vi "PH_gentec_P-Link.Action Measure.vi"(0 "VI in":refnum<vi>, 5 "error in (no error)":errorcluster) -> (14 "VI out":refnum<vi>, 19 "error out":errorcluster)   [LabVIEW 2014, in "PH_gentec_P-Link.lvlib"]
uses:
  PH_gentec_P-Link.lvlib
  PH_Basics/PH_Powermeter_BaseClass/PH_Powermeter_BaseClass.State.ctl
  PH_Basics/PH_Powermeter_BaseClass/PH_Powermeter_BaseClass.lvlib
  instr.lib/Gentec-P-Link/gentec-P-Link - Driver.lvlib
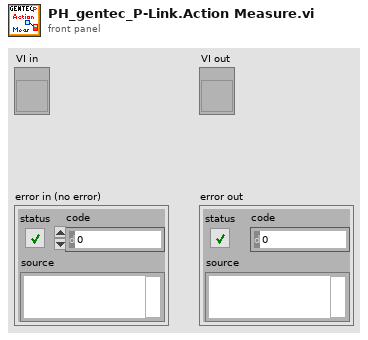
[diagram p1: front panel]
types:
  T1 = typedef "PH_Powermeter_BaseClass.lvlib/PH_Powermeter_BaseClass.State.ctl" = enum32{"off", "operating", "opened", "checked", "connected", "Sets to change", "running"}
  T2 = typedef "PH_Powermeter_BaseClass.lvlib/PH_Powermeter_BaseClass.i attribute.ctl" = cluster{"GUI References":T3, "Connection":T4, "Head Attributes":T5, "VISA resource":refnum<visa-resource-name>, "Energy":T6, "Service ID Energy":i32, "Wanted Settings":T7, "Current Settings":T7}
  T3 = typedef "PH_Powermeter_BaseClass.lvlib/PH_Powermeter_BaseClass.GUI Refs.ctl" = cluster{"Head Attributes":refnum<vi>, "Energy":refnum<vi>, "Connection":refnum<vi>, "VISA Resource":refnum<vi>, "Scaling Factor":refnum<vi>, "Range":refnum<vi>, "Wavelength":refnum<vi>, "Trigger Level":refnum<vi>, "Wanted Settings":refnum<vi>, "Current Settings":refnum<vi>}
  T4 = typedef "PH_Powermeter_BaseClass.lvlib/PH_Powermeter_BaseClass.Connection.ctl" = cluster{"failed checks":i8, "Timeout":bool, "Data read":string, "Failure":bool, "Error":bool, "State":T1}
  T5 = typedef "PH_Powermeter_BaseClass.lvlib/PH_Powermeter_BaseClass.Head Attributes.ctl" = cluster{"Instrument Type":string, "Head Version":string, "Head Name":string, "Serial Number":string, "Firmware":string, "Sensor Type":string, "MinimumRange":u32, "Maximum Range":u32, "Min Wavelength":i32, "Max Wavelength":i32}
  T6 = typedef "PH_Powermeter_BaseClass.lvlib/PH_Powermeter_BaseClass.Energy.ctl" = cluster{"current Value":dbl, "unscaled":dbl, "Scaling Factor":dbl}
  T7 = typedef "PH_Powermeter_BaseClass.lvlib/PH_gentec_BaseClass.Head Settings.ctl" = cluster{"Trigger Level":dbl, "Wavelength":u32, "Range":u32}
  T8 = typedef "PH_gentec_P-Link.lvlib/PH_gentec_P-Link.i attribute.ctl" = cluster{"GUI References":cluster{"Wanted Head Settings":refnum<vi>, "Current Head Settings":refnum<vi>, "Set Auto Range":refnum<vi>, "Trigger Polarity":refnum<vi>, "Trigger Source":refnum<vi>, "Waveform Averages":refnum<vi>, "Continuous":refnum<vi>, "get one Value":refnum<vi>}, "Wanted Head Settings":T9, "Current Head Settings":T9}
  T9 = typedef "PH_gentec_P-Link.lvlib/PH_gentec_P-Link.Head Settings.ctl" = cluster{"Measurement Mode":T10, "Enable Anticipation":bool, "Set Auto Range":bool, "Block Signal":bool, "Set Head Attenuator":bool, "Enable SSE":bool, "Trigger Polarity":T11, "Trigger Source":T12, "Waveform Averages":T13, "Set Zero":i32, "Current":i32, "Start Data Flow":bool}
  T10 = typedef "gentec-M-Link - Driver.lvlib/gentec-M-Link.Measurement Mode.ctl" = u16
  T11 = typedef "gentec-M-Link - Driver.lvlib/gentec-M-Link.Trigger Polarity.ctl" = u16
  T12 = typedef "gentec-M-Link - Driver.lvlib/gentec-M-Link.Trigger Source.ctl" = u16
  T13 = typedef "gentec-M-Link - Driver.lvlib/gentec-M-Link.Waveform Averages.ctl" = u16
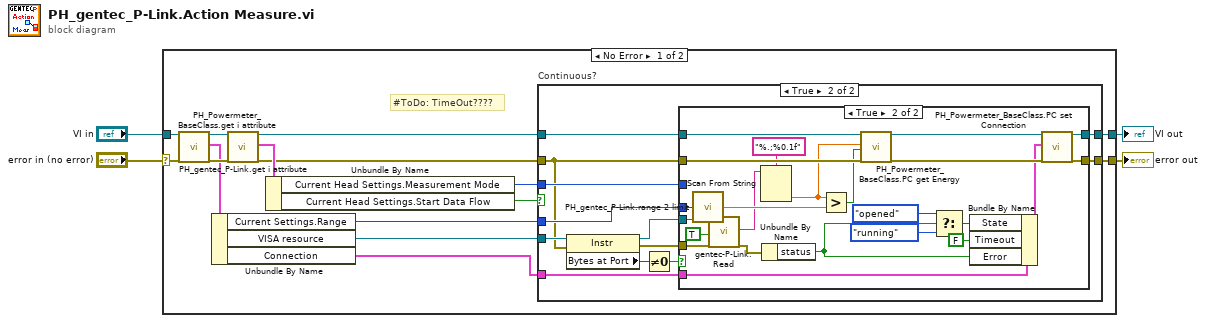
[diagram p0: block diagram]
diagram:
  n1 = case shown="No Error" "error in (no error)" {
    selector: "error in (no error)" -> [w6 w59]
    tunnel: [w14 w60] -> w4
    tunnel: [w13 w59] -> w3
    tunnel: "VI in" -> [w11 w60]
    frame No Error {
      # "#ToDo: TimeOut????"
      n2 = call "PH_Powermeter_BaseClass.get i attribute.vi"("i ref in"=w11, "error in (no error)"=w6) -> ("i ref out"=w10:refnum<vi>, "i attribute"=w9:T2, "error out"=w12:errorcluster)  [unwired: 15 in]
      n3 = Unbundle By Name(w9) -> ("Current Settings.Range"=w5:u32, "VISA resource"=w8:refnum<visa-resource-name>, "Connection"=w7:T4)
      n4 = call "PH_gentec_P-Link.get i attribute.vi"("i ref in"=w10, "error in (no error)"=w12) -> ("i ref out"=w17:refnum<vi>, "i attribute"=w18:T8, "error out"=w16:errorcluster)  [unwired: 15 in]
      n5 = Unbundle By Name(w18) -> ("Current Head Settings.Measurement Mode"=w19:T10, "Current Head Settings.Start Data Flow"=w15:bool)
      n6 = case "Continuous?" shown="True" w15 {
        tunnel: w17 -> [w21 w26]
        tunnel: [w21 w24] -> w14
        tunnel: w16 -> [w20 w25]
        tunnel: [w20 w23] -> w13
        tunnel: w8 -> [_ w29]
        tunnel: w19 -> [_ w28]
        tunnel: w5 -> [_ w27]
        tunnel: w7 -> [_ w22]
        frame False {
        }
        frame True {
          n7 = property class="Instr"(reference=w29, error in=w25) -> (reference out=w31:refnum<visa-resource-name>, error out=w30:errorcluster, "Bytes at Port"=w33:u32)
          n8 = Not Equal To 0?(x=w33) -> (x != 0?=w32:bool)
          n9 = case shown="True" w32 {
            tunnel: w31 -> [_ w42]
            tunnel: w30 -> [_ w41]
            tunnel: w28 -> [_ _]
            tunnel: w25 -> [w35 w58]
            tunnel: [w35 w50] -> w23
            tunnel: w26 -> [w34 w57]
            tunnel: [w34 w52] -> w24
            tunnel: w27 -> [_ w54]
            tunnel: w22 -> [_ w49]
            frame False {
            }
            frame True {
              n10 = call "PH_gentec_P-Link.range 2 limit.vi"("Range"=w54) -> ("limit"=w56:dbl)
              n11 = call "gentec-P-Link.Read.vi"("VISA resource name"=w42, "ReadOneByOne?"=TRUE, "error in (no error)"=w41) -> ("Read Buffer"=w38:string, "error out"=w40:errorcluster)  [unwired: 13 in, 2 out]
              n12 = Scan From String(format string="%.;%0.1f", input string=w38) -> (output 1=w37:dbl)  [unwired: 3 in, 3 out]
              n13 = Unbundle By Name(w40) -> ("status"=w47:bool)
              n14 = Greater?(x=w37, y=w56) -> (0:w55:bool)
              n15 = call "PH_Powermeter_BaseClass.PC get Energy.vi"("i ref in"=w57, "unscaled Energy [J]"=w37, "Out of range?"=w55, "error in"=w58) -> ("i ref out"=w53:refnum<vi>, "error out"=w51:errorcluster)  [unwired: 14 in]
              n16 = Select(t=PH_Powermeter_BaseClass.State."opened", s=w47, f=PH_Powermeter_BaseClass.State."running" ("State")) -> (s? t:f=w45:T1)
              n17 = Bundle By Name(cluster=w49, "State"=w45, "Timeout"=FALSE, "Error"=w47) -> (w48:T4)
              n18 = call "PH_Powermeter_BaseClass.PC set Connection.vi"("VI in"=w53, "Connection"=w48, "error in (no error)"=w51) -> ("VI out"=w52:refnum<vi>, "error out"=w50:errorcluster)  [unwired: 15 in]
            }
          }
        }
      }
    }
    frame Error {
    }
  }
  "VI out" <- w4
  "error out" <- w3
